vi "GetLogo.vi"(7 "LabVIEW Web Service Request":refnum<class "Web Request.lvclass">) -> ()   [LabVIEW 2013]
uses:
  <vilib>/wsapi/Web Request.lvclass
panel:
  # "Use the Web Service Request input terminal to call the VIs on the Web Services palette. Do not remove it from the connector pane unless you don't need access to the palette."
  # "Each additional control wired to the connector pane will be available as an input in the URL. To include an indicator in terminal-mode output (the default setting), it must also be wired to the connector pane."
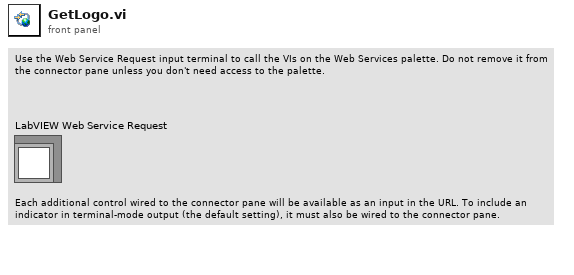
[diagram p1: front panel]
types:
  T1 = typedef "imagedata.ctl" = cluster{"image type":i32, "image depth":i32, "image":u8[], "mask":u8[], "colors":u32[], "Rectangle":cluster{"left":i16, "top":i16, "right":i16, "bottom":i16}}
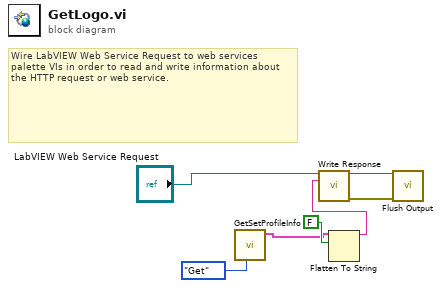
[diagram p0: block diagram]
diagram:
  # "Wire LabVIEW Web Service Request to web services palette VIs in order to read and write information about the HTTP request or web service."
  n1 = call "GetSetProfileInfo.vi"("Get/Set State"=enum16{"Get", "Set", "Load"}."Get") -> ("image data out"=w2:T1)  [unwired: 8 in, 2 out]
  n2 = Flatten To String(anything=w2, prepend array or string size? (T)=FALSE) -> (data string=w7:string)  [unwired: 2 in, 2 out]
  n3 = call <vilib>:"Write Response.vi"("LabVIEW Web Service Request"="LabVIEW Web Service Request", "response string"=w7) -> ("LabVIEW Web Service Request out"=w4:refnum<class "Web Request.lvclass">, "error out"=w5:errorcluster)  [unwired: 12 in]
  n4 = call <vilib>:"Flush Output.vi"("LabVIEW Web Service Request"=w4, "error in (no error)"=w5) -> ()  [unwired: 12 in, 2 out]
